vi "Read Ref.vi"(8 "error in (no error)":errorcluster, 11 "OSA200 in":refnum<class "OSA200.lvclass">) -> (0 "error out":errorcluster, 2 "Ref":u32, 3 "OSA200 out":refnum<class "OSA200.lvclass">)   [LabVIEW 2010, in "OSA200.lvclass"]
uses:
  OSA200.lvclass
  OSA200.lvclass/OSA200.ctl
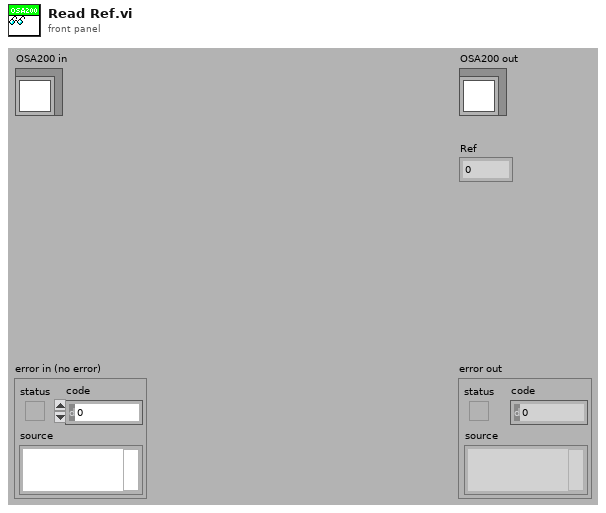
[diagram p1: front panel]
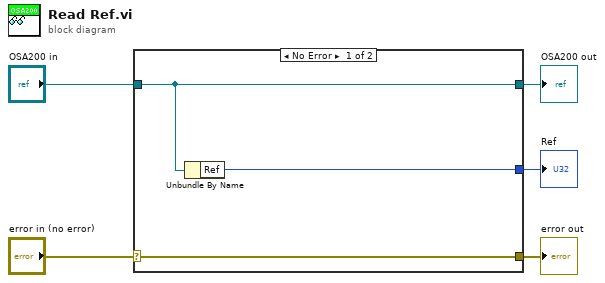
[diagram p0: block diagram]
diagram:
  n1 = case shown="No Error" "error in (no error)" {
    selector: "error in (no error)" -> [w8 w9]
    tunnel: [w8 w9] -> w4
    tunnel: [w7 w10] -> w2
    tunnel: "OSA200 in" -> [w7 w10]
    tunnel: [w6 _] -> w1
    frame No Error {
      n2 = Unbundle By Name(w7) -> ("Ref"=w6:u32)
    }
    frame Error {
    }
  }
  "error out" <- w4
  "OSA200 out" <- w2
  "Ref" <- w1
